vi "Save IMG.vi"(4 "Comment":string, 5 "file path":path, 6 "Image":T2, 7 "ROI Descriptor":T1) -> ()   [LabVIEW 2016]
doc: "10/1/98\nSave IMG.vi\nJim Yagmin\n\n This VI allows a user to save a whole image (default) or outline and save an ROI of an image (in rectangle form) as an external .IMG file, readable by Protox and SDP. Kernel images (.IMG) are useful for cutting out the \"empty spaces\" that affect the histogram graph when trying to specify an ideal contrast for a sequence.\n This subVI is organized in a four-step sequence that appends information to the .IMG file. First the \"IM\" header is added to the new file, then the numeric information is appended (comment lenght, width, height, etc.). Next, the comment and reserved space are appended to the file and, finally, the ROI-specified segment of the image is attached and the .IMG file is saved.\n This subVI follows the format of .IMG as specified on page C-2 in Appendix C of Itex 150/151 Programmer's Manual, Part II. This is the .IMG file format:\n\nBytes Contents\n0-1 Characters \"IM\" indicate this is an image file\n2-3 Comment length (maximum 255)\n4-5 Width of the image in pixels\n6-7 Height of the image in lines\n8-9 Coordinates of original X-axis (horizontal) position\n10-11 Coordinates of original Y-axis (vertical) position\n12-13 File type flag:\n 0 = EIGHT_BIT (What we use)\n 1 = COMPRESSED\n 4 = SIXTEEN_BIT\n14-63 Reserved\n64-n Comment area - variable in length, 255 bytes max.\nn-m Data area - one byte per pixel stored in row order, from the top\n to the bottom of the image (compressed or not)\n UNCOMPRESSED - One byte per pixel stored in row order\n SIXTEEN_BIT - Two bytes per pixel\n\n .IMG format also requires an archaic byte structure, which is why in Frame 2 of the Sequence structure there is a big mess of conversions. The appendix goes on to describe the problem as such:\n\nByte Swapping and Image, LUT Files\n Headers in image and Look-Up Table (LUT) files are stored in the native host byte ordering scheme. Keep this in mind when transporting images or LUT files from one system to another or problems may arise.\n On the IBM AT for example, a 16-bit number is stored with its least significant byte first, followed by its most significant byte. On a Motorola 68000 based system, the bytes are reversed or swapped.\n\n This problem can be seen if you look at an .IMG file using a hex editing program (such as Hexedit). The correct format is:\n\n49 4D 19 00 ... where \"49 4D\" stands for the initial \"IM\" and the\n\"19 00\" is the first 16-bit number, the comment length. What Labview produces, though is the following:\n\n49 4D 00 19 ... which is why all the swapping stuff is necessary."
uses:
  <vilib>/vision/Image Controls.llb/IMAQ Image.ctl
panel:
  out "Global Rectangle":i32[](array[numeric])
  # "x1Left"
  # "y1Top"
  # "x2Right"
  # "y2Bottom"
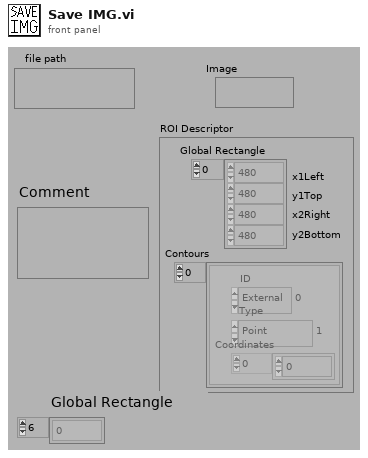
[diagram p1: front panel]
types:
  T1 = cluster{"Global Rectangle":i32[], "Contours":cluster{"ID":enum32{"External", "Internal"}, "Type":enum32{"No Selection", "Point", "Line", "Rectangle", "Oval", "Polygon", "Free", "Unused1", "Unused2", "Unused3", "Broken Line", "Free Hand Line"}, "Coordinates":i32[]}[]}
  T2 = typedef "IMAQ Image.ctl" = refnum<image>
  T3 = enum16{"open", "open or create", "create or replace", "create"}
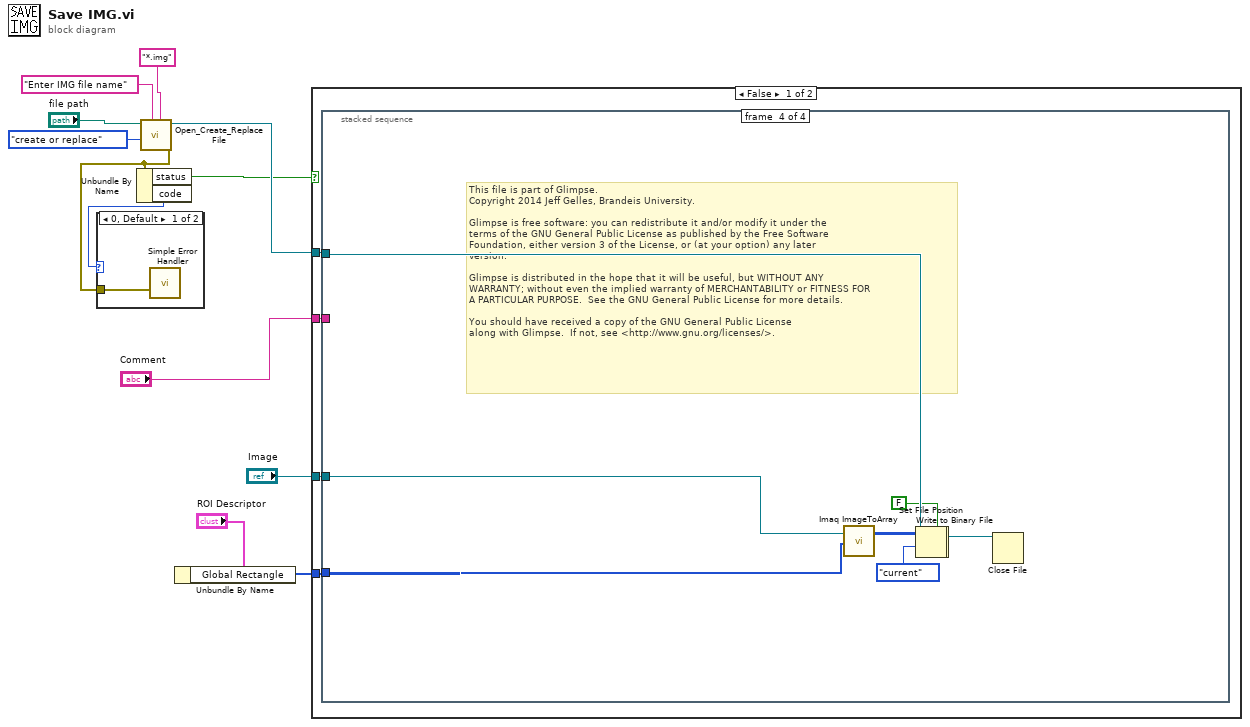
[diagram p0: block diagram]
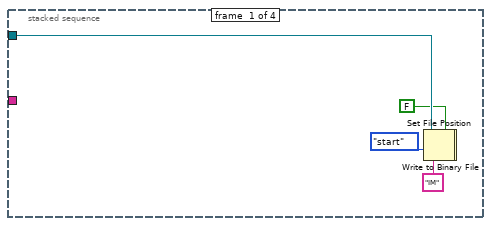
[diagram p2: hidden frame]
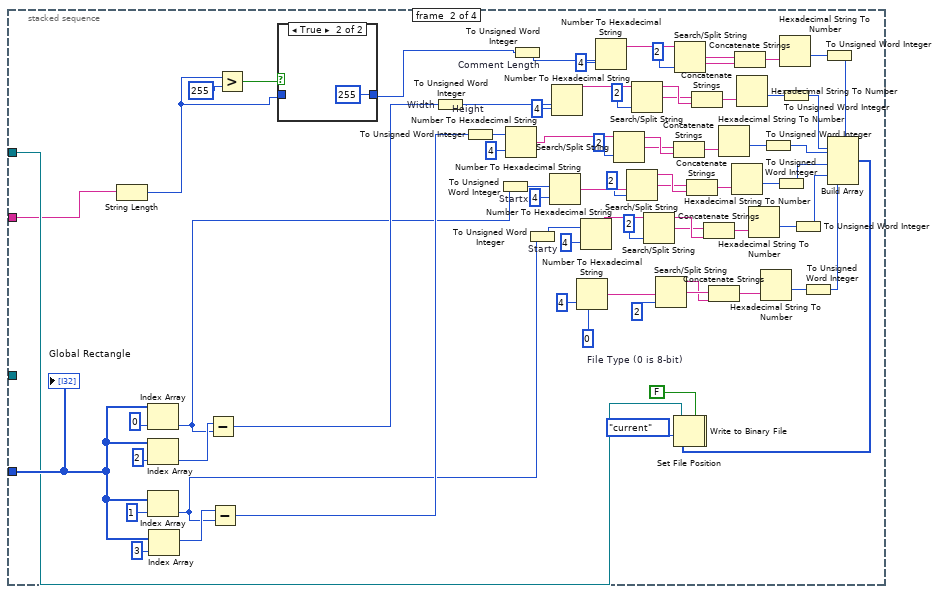
[diagram p3: hidden frame]
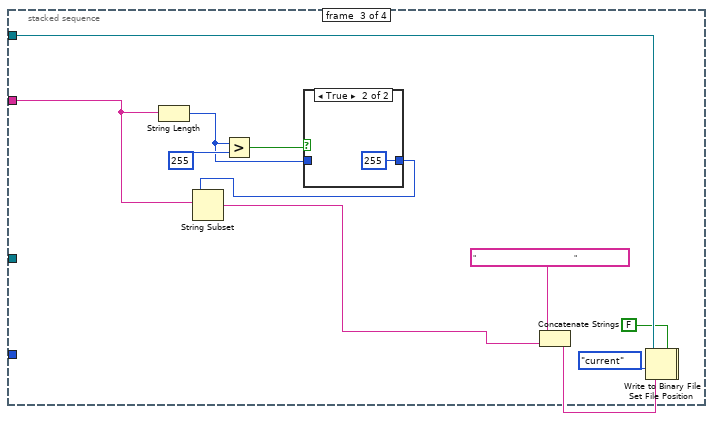
[diagram p5: hidden frame]
diagram:
  # "This file is part of Glimpse. \nCopyright 2014 Jeff Gelles, Brandeis University.    \n\nGlimpse is free software: you can redistribute it and/or modify it under the \nterms of the GNU General Public License as published by the Free Software \nFoundation, either version 3 of the License, or (at your option) any later \nversion.\n\nGlimpse is distributed in the hope that it will be useful, but WITHOUT ANY \nWARRANTY; without even the implied warranty of MERCHANTABILITY or FITNESS FOR \nA PARTICULAR PURPOSE.  See the GNU General Public License for more details.\n\nYou should have received a copy of the GNU General Public License\nalong with Glimpse.  If not, see <http://www.gnu.org/licenses/>."
  n1 = call <vilib>:"Open_Create_Replace File.vi"("pattern"="*.img", "prompt"="Enter IMG file name", "function (open:0)"=T3."create or replace", "file path"="file path") -> ("error out"=w7:errorcluster, "refnum"=w3:refnum<file>)  [unwired: 3 in, 3 out]
  n2 = Unbundle By Name(w7) -> ("status"=w1:bool, "code"=w8:i32)
  n3 = case shown="0, Default" w8 {
    tunnel: w7 -> [w13 _]
    frame 0, Default {
      n4 = call <vilib>:"Simple Error Handler.vi"("error in (no error)"=w13) -> ()  [unwired: 1 in, 8 out]
    }
    frame 43 {
    }
  }
  n5 = Unbundle By Name("ROI Descriptor") -> ("Global Rectangle"=w11:i32[])
  n6 = case shown="False" w1 {
    tunnel: w11 -> [w17 _]
    tunnel: "Comment" -> [w16 _]
    tunnel: "Image" -> [w15 _]
    tunnel: w3 -> [w14 _]
    frame False {
      n7 = stacked-sequence {
        tunnel: w17 -> [_ w93 _ w125]
        tunnel: w14 -> [w21 w91 w107 w123]
        tunnel: w16 -> [_ w90 w110 _]
        tunnel: w15 -> [_ _ _ w120]
        frame #0 {
          n8 = Set File Position(refnum=w21, from (0:start)=enum16{"start", "end", "current"}."start" ("pos mode (0:2)")) -> (refnum out=w20:refnum<file>, error out=w19:errorcluster)  [unwired: 1 in, 1 out]
          n9 = Write to Binary File(file (use dialog)=w20, data="IM", error in=w19, 5:FALSE ("prepend array or string size? (T)")) -> ()  [unwired: 5 out]
        }
        frame #1 {
          w35 = 0  # File Type (0 is 8-bit)
          n10 = String Length ("Comment Length")(string=w90) -> (length=w28:i32)
          n11 = Index Array(array=w93, index=0) -> (element=w32:i32)
          n12 = Index Array(array=w93, index=2) -> (element=w95:i32)
          n13 = Index Array(array=w93, index=1) -> (element=w31:i32)
          n14 = Index Array(array=w93, index=3) -> (element=w94:i32)
          n15 = Subtract(x=w95, y=w32) -> (x-y=w34:i32)
          n16 = Subtract(x=w94, y=w31) -> (x-y=w33:i32)
          n17 = Greater?(x=w28, y=255) -> (0:w29:bool)
          n18 = case shown="True" w29 {
            tunnel: w28 -> [w100 _]
            tunnel: [w100 255] -> w27
            frame False {
            }
            frame True {
            }
          }
          n19 = To Unsigned Word Integer "Width"(number=w34) -> (unsigned 16bit integer=w87:u16)
          n20 = To Unsigned Word Integer "Height"(number=w33) -> (unsigned 16bit integer=w86:u16)
          n21 = To Unsigned Word Integer "Startx"(number=w32) -> (unsigned 16bit integer=w85:u16)
          n22 = Number To Hexadecimal String(1:i16 4 ("width (-)"), 2:w86) -> (0:w65:string)
          n23 = To Unsigned Word Integer "Comment Length"(number=w27) -> (unsigned 16bit integer=w88:u16)
          n24 = To Unsigned Word Integer "Starty"(number=w31) -> (unsigned 16bit integer=w84:u16)
          n25 = Number To Hexadecimal String(1:i16 4 ("width (-)"), 2:w85) -> (0:w59:string)
          n26 = Number To Hexadecimal String(1:i16 4 ("width (-)"), 2:w87) -> (0:w72:string)
          n27 = Number To Hexadecimal String(1:i16 4 ("width (-)"), 2:w35) -> (0:w45:string)
          n28 = Number To Hexadecimal String(1:i16 4 ("width (-)"), 2:w84) -> (0:w51:string)
          n29 = Number To Hexadecimal String(1:i16 4 ("width (-)"), 2:w88) -> (0:w83:string)
          n30 = Search/Split String(string=w65, offset (0)=2) -> (substring before match=w69:string, match + rest of string=w68:string)  [unwired: 2 out]
          n31 = Search/Split String(string=w59, offset (0)=2) -> (substring before match=w63:string, match + rest of string=w62:string)  [unwired: 2 out]
          n32 = Search/Split String(string=w72, offset (0)=2) -> (substring before match=w76:string, match + rest of string=w75:string)  [unwired: 2 out]
          n33 = Search/Split String(string=w51, offset (0)=2) -> (substring before match=w55:string, match + rest of string=w54:string)  [unwired: 2 out]
          n34 = Search/Split String(string=w45, offset (0)=2) -> (substring before match=w42:string, match + rest of string=w48:string)  [unwired: 2 out]
          n35 = Concatenate Strings(w68, w69) -> (w67:string)
          n36 = Set File Position(refnum=w91, from (0:start)=enum16{"start", "end", "current"}."current" ("pos mode (0:2)")) -> (refnum out=w26:refnum<file>, error out=w25:errorcluster)  [unwired: 1 in, 1 out]
          n37 = Search/Split String(string=w83, offset (0)=2) -> (substring before match=w81:string, match + rest of string=w80:string)  [unwired: 2 out]
          n38 = Concatenate Strings(w62, w63) -> (w61:string)
          n39 = Concatenate Strings(w75, w76) -> (w74:string)
          n40 = Concatenate Strings(w54, w55) -> (w53:string)
          n41 = Concatenate Strings(w48, w42) -> (w47:string)
          n42 = Hexadecimal String To Number(string=w67) -> (number=w66:u32)  [unwired: 3 out]
          n43 = Hexadecimal String To Number(string=w61) -> (number=w60:u32)  [unwired: 3 out]
          n44 = Concatenate Strings(w80, w81) -> (w79:string)
          n45 = Hexadecimal String To Number(string=w74) -> (number=w73:u32)  [unwired: 3 out]
          n46 = Hexadecimal String To Number(string=w53) -> (number=w52:u32)  [unwired: 3 out]
          n47 = Hexadecimal String To Number(string=w47) -> (number=w46:u32)  [unwired: 3 out]
          n48 = To Unsigned Word Integer(number=w66) -> (unsigned 16bit integer=w64:u16)
          n49 = To Unsigned Word Integer(number=w60) -> (unsigned 16bit integer=w56:u16)
          n50 = Hexadecimal String To Number(string=w79) -> (number=w78:u32)  [unwired: 3 out]
          n51 = To Unsigned Word Integer(number=w73) -> (unsigned 16bit integer=w71:u16)
          n52 = To Unsigned Word Integer(number=w52) -> (unsigned 16bit integer=w49:u16)
          n53 = To Unsigned Word Integer(number=w46) -> (unsigned 16bit integer=w43:u16)
          n54 = To Unsigned Word Integer(number=w78) -> (unsigned 16bit integer=w77:u16)
          n55 = Build Array(w77, w71, w64, w56, w49, w43) -> (w89:u16[])
          n56 = Write to Binary File(file (use dialog)=w26, data=w89, error in=w25, 5:FALSE ("prepend array or string size? (T)")) -> ()  [unwired: 5 out]
          "Global Rectangle" <- w93
        }
        frame #2 {
          n57 = String Length(string=w110) -> (length=w106:i32)
          n58 = Greater?(x=w106, y=255) -> (0:w114:bool)
          n59 = case shown="True" w114 {
            tunnel: w106 -> [w115 _]
            tunnel: [w115 255] -> w112
            frame False {
            }
            frame True {
            }
          }
          n60 = String Subset(string=w110, length (rest)=w112) -> (substring=w109:string)  [unwired: 1 out]
          n61 = Concatenate Strings("                                                 ", w109) -> (w105:string)
          n62 = Set File Position(refnum=w107, from (0:start)=enum16{"start", "end", "current"}."current" ("pos mode (0:2)")) -> (refnum out=w104:refnum<file>, error out=w103:errorcluster)  [unwired: 1 in, 1 out]
          n63 = Write to Binary File(file (use dialog)=w104, data=w105, error in=w103, 5:FALSE ("prepend array or string size? (T)")) -> ()  [unwired: 5 out]
        }
        frame #3 {
          n64 = call "Imaq ImageToArray"("Optional Rectangle"=w125, "Image"=w120) -> ("Image Pixels (U8)"=w122:u8[][])  [unwired: 1 in, 5 out]
          n65 = Set File Position(refnum=w123, from (0:start)=enum16{"start", "end", "current"}."current" ("pos mode (0:2)")) -> (refnum out=w119:refnum<file>, error out=w118:errorcluster)  [unwired: 1 in, 1 out]
          n66 = Write to Binary File(file (use dialog)=w119, data=w122, error in=w118, 5:FALSE ("prepend array or string size? (T)")) -> (refnum out=w121:refnum<file>)  [unwired: 4 out]
          n67 = Close File(refnum=w121) -> ()  [unwired: 1 in, 2 out]
        }
      }
    }
    frame True {
    }
  }
